vi "get data name.vi"(1 "data in":variant) -> (0 "Name":string)   [LabVIEW 2023, in "Publisher Subscriber.lvlib"]
uses:
  <userlib>/_Publisher Subscriber/Publisher Subscriber.lvlib
  <vilib>/Utility/Data Type/NI_Data Type.lvlib
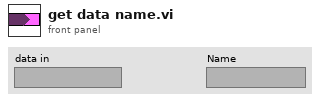
[diagram p1: front panel]
types:
  T1 = typedef "NI_Data Type.lvlib/Data Type.ctl" = enum8{"Invalid Type", "Void", "I8", "I16", "I32", "I64", "U8", "U16", "U32", "U64", "Single Float", "Double Float", "Extended Float", "Single Complex", "Double Complex", "Extended Complex", "Enum U8", "Enum U16", "Enum U32", "Enum U64", "Single Float With Unit", "Double Float With Unit", "Extended Float With Unit", "Single Complex with Unit", "Double Complex with Unit", "Extended Complex with Unit", "Boolean", "String", "Path", "Picture", "Tag", "Array", "Cluster", "Variant", "LV Variant", "Waveform", "Timestamp", "Digital Waveform", "Digital Data", "ExpressData", "Refnum", "External Data", "VI", "Poly VI", "LabVIEW Class Instance", "Fixed Point", "Set Collection", "Map Collection"}
  T2 = typedef "NI_Data Type.lvlib/Type Definition Info.ctl" = cluster{"Name":string, "Timestamp":u32}
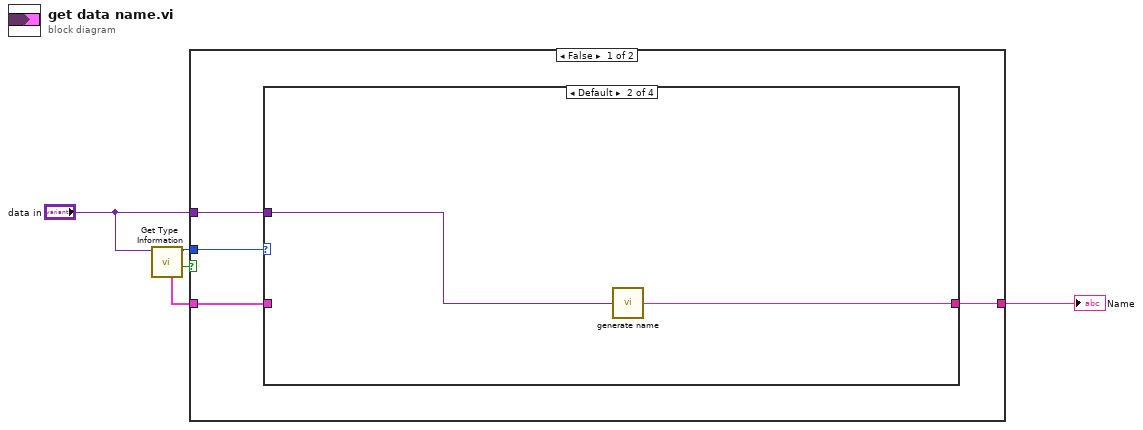
[diagram p0: block diagram]
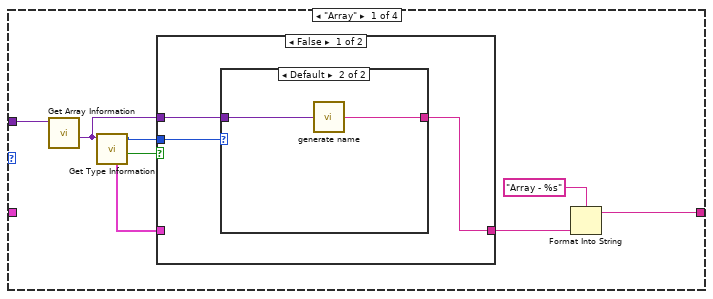
[diagram p2: hidden frame]
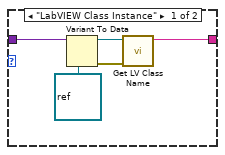
[diagram p3: hidden frame]
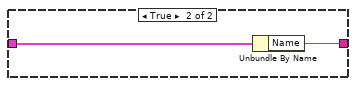
[diagram p4: hidden frame]
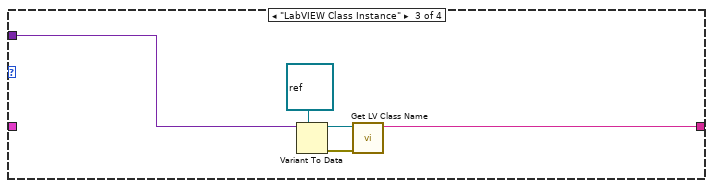
[diagram p5: hidden frame]
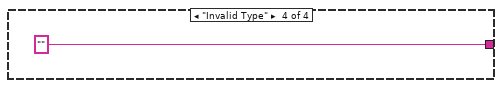
[diagram p6: hidden frame]
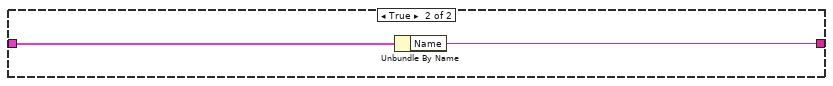
[diagram p7: hidden frame]
diagram:
  n1 = call <vilib>:"Get Type Information.vi"("variant"="data in") -> ("type definition"=w1:bool, "type"=w5:T1, "type definition info"=w2:T2)  [unwired: 6 in, 2 out]
  n2 = case shown="False" w1 {
    tunnel: w2 -> [w6 w39]
    tunnel: [w8 w38] -> w3
    tunnel: "data in" -> [w7 _]
    tunnel: w5 -> [w9 _]
    frame False {
      n3 = case shown="Default" w9 {
        tunnel: [w10 w30 w33 "" ("Name")] -> w8
        tunnel: w7 -> [w17 w31 w34 _]
        tunnel: w6 -> [_ _ _ _]
        frame "Array" {
          n4 = call <vilib>:"Get Array Information.vi"("variant"=w17) -> ("array element data type"=w13:variant)  [unwired: 7 in, 3 out]
          n5 = call <vilib>:"Get Type Information.vi"("variant"=w13) -> ("type definition"=w16:bool, "type"=w14:T1, "type definition info"=w15:T2)  [unwired: 6 in, 2 out]
          n6 = case shown="False" w16 {
            tunnel: w15 -> [_ w29]
            tunnel: [w19 w28] -> w11
            tunnel: w14 -> [w18 _]
            tunnel: w13 -> [w20 _]
            frame False {
              n7 = case shown="Default" w18 {
                tunnel: w20 -> [w23 w27]
                tunnel: [w22 w26] -> w19
                frame "LabVIEW Class Instance" {
                  n8 = Variant To Data(type=refnum<class> refnum ("LabVIEW Object"), Variant=w23) -> (data=w24:refnum<class>, error out=w21:errorcluster)  [unwired: 1 in]
                  n9 = call <vilib>:"Get LV Class Name.vi"("error in (no error)"=w21, "object"=w24) -> ("class name"=w22:string)  [unwired: 8 in, 1 out]
                }
                frame Default {
                  n10 = call <userlib>:"generate name.vi"("variant"=w27) -> ("name"=w26:string)
                }
              }
            }
            frame True {
              n11 = Unbundle By Name(w29) -> ("Name"=w28:string)
            }
          }
          n12 = Format Into String(format string="Array - %s", w11) -> (resulting string=w10:string)  [unwired: 2 in, 1 out]
        }
        frame Default {
          n13 = call <userlib>:"generate name.vi"("variant"=w31) -> ("name"=w30:string)
        }
        frame "LabVIEW Class Instance" {
          n14 = Variant To Data(type=refnum<class> refnum ("LabVIEW Object"), Variant=w34) -> (data=w35:refnum<class>, error out=w32:errorcluster)  [unwired: 1 in]
          n15 = call <vilib>:"Get LV Class Name.vi"("error in (no error)"=w32, "object"=w35) -> ("class name"=w33:string)  [unwired: 8 in, 1 out]
        }
        frame "Invalid Type" {
        }
      }
    }
    frame True {
      n16 = Unbundle By Name(w39) -> ("Name"=w38:string)
    }
  }
  "Name" <- w3
